vi "CD Read Engine_Parse Message.vi"(8 "Error (in)":errorcluster, 9 "Inline Status Channels Refs":T1[](array[typedef]) format="%.0x", 10 "Record []":T11[](array[typedef]) {"type" format="%04x"; "activity" format="%04x"; "error" format="%04x"; "cwd1" format="%04x"; "cwd2" format="%04x"; "swd1" format="%04x"; "swd2" format="%04x"; "data" format="%04x"}, 11 "RT Inline Data_Data Description_Channels":T2[](array[typedef]) {"Frame Drescriptors"."RT"."Status Channel Ref" format="%.0x"; "Frame Drescriptors"."RT"."Words Block Data Refs"."Data Reference" format="%.0x"; "Frame Drescriptors"."RT"."Timestamp Channel Data Reference" format="%.0x"; "Frame Drescriptors"."BC"."Status Channel Refs" format="%.0x"; "Frame Drescriptors"."BC"."Words Block Data Refs"."Data Reference" format="%.0x"; "Frame Drescriptors"."BC"."Timestamp Channel Data Reference" format="%.0x"}) -> (0 "Error (out)":errorcluster)   [LabVIEW 2020, in "Ballard MIL-1553 Engine.lvlib"]
uses:
  Ballard MIL-1553 Engine.lvlib
  <instrlib>/BTICardLib/Public/Controls/1553 Record.ctl
  Controls/RT Inline Data_Data Description_Channel.ctl
  Controls/RT Inline Frame Descriptor.ctl
  Controls/RT Inline Frame Descriptor_BC.ctl
  <vilib>/NI VeriStand/Custom Device API/Data Reference.ctl
  <vilib>/NI VeriStand/Custom Device API/Block Data Reference.ctl
  <vilib>/NI VeriStand/Custom Device API/Custom Device Item Ref.ctl
  Controls/RT Inline Frame Descriptor_RT.ctl
  Shared/Controls and Global/RT CWD2.ctl
  Shared/Controls and Global/RT CWD1.ctl
  Shared/Controls and Global/RT messageType.ctl
  <vilib>/NI VeriStand/Custom Device Tools/Custom Device Utility Library/Custom Device Utility Library.lvlib
  Shared/Ballard 1553 Shared.lvlib
  <vilib>/NI VeriStand/Custom Device API/Custom Device API.lvlib
  <instrlib>/BTICardLib/BTICardLV.lvlib
panel:
  out "Physical Channel":u16
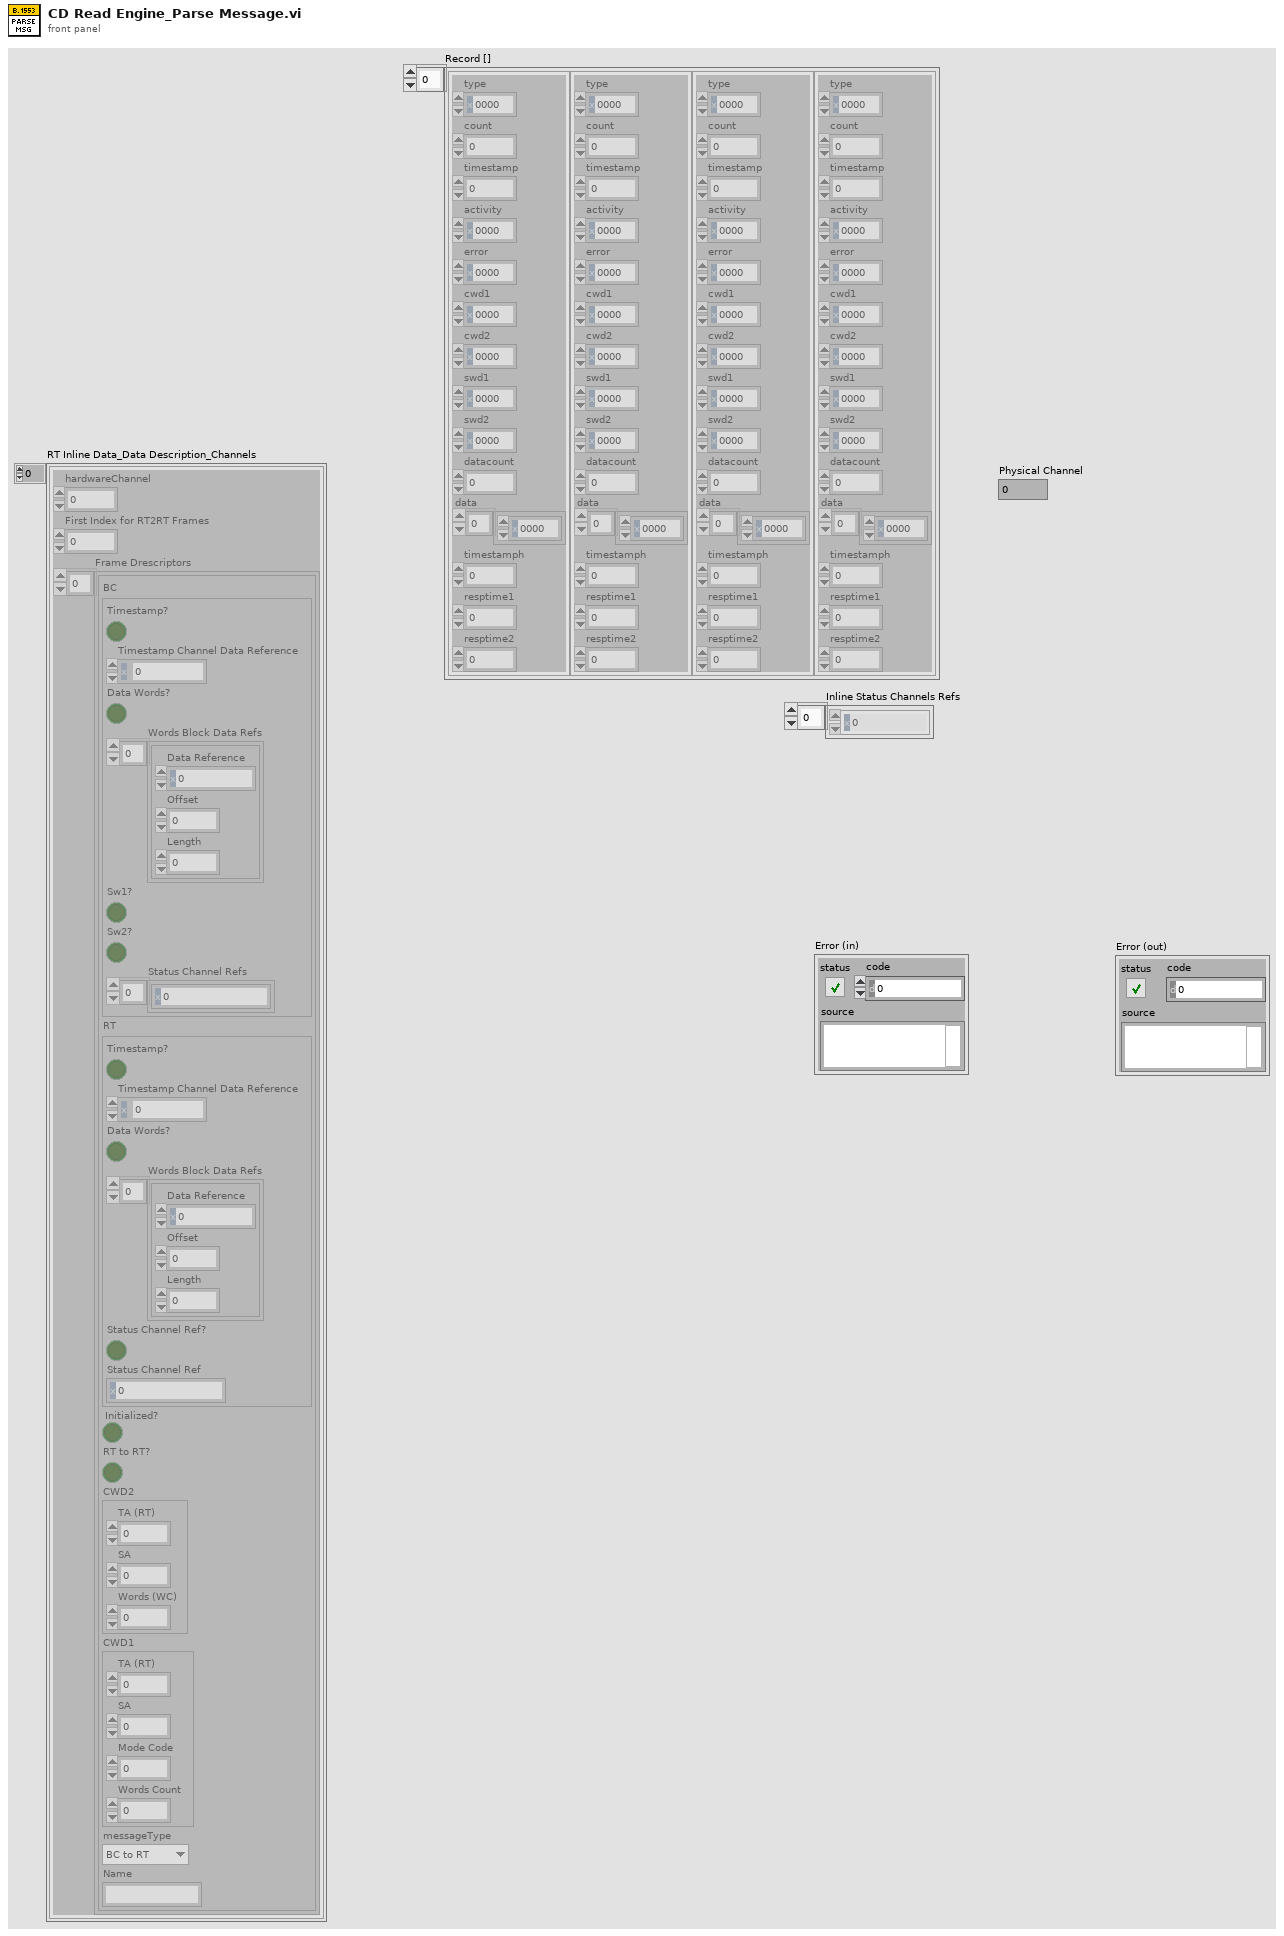
[diagram p1: front panel]
types:
  T1 = typedef "Custom Device API.lvlib/Data Reference.ctl" = i32
  T2 = typedef "Ballard MIL-1553 Engine.lvlib/RT Inline Data_Data Description_Channel.ctl" = cluster{"hardwareChannel":u16, "First Index for RT2RT Frames":i32, "Frame Drescriptors":T3[]}
  T3 = typedef "Ballard MIL-1553 Engine.lvlib/RT Inline Frame Descriptor.ctl" = cluster{"BC":T4, "RT":T7, "Initialized?":bool, "RT to RT?":bool, "CWD2":T8, "CWD1":T9, "messageType":T10, "Name":string}
  T4 = typedef "Ballard MIL-1553 Engine.lvlib/RT Inline Frame Descriptor_BC.ctl" = cluster{"Timestamp?":bool, "Timestamp Channel Data Reference":T1, "Data Words?":bool, "Words Block Data Refs":T5[], "Sw1?":bool, "Sw2?":bool, "Status Channel Refs":T6[]}
  T5 = typedef "Custom Device API.lvlib/Block Data Reference.ctl" = cluster{"Data Reference":T1, "Offset":u64, "Length":u64}
  T6 = typedef "Custom Device API.lvlib/Custom Device Item Ref.ctl" = u64
  T7 = typedef "Ballard MIL-1553 Engine.lvlib/RT Inline Frame Descriptor_RT.ctl" = cluster{"Timestamp?":bool, "Timestamp Channel Data Reference":T1, "Data Words?":bool, "Words Block Data Refs":T5[], "Status Channel Ref?":bool, "Status Channel Ref":T6}
  T8 = typedef "Ballard 1553 Shared.lvlib/RT CWD2.ctl" = cluster{"TA (RT)":i8, "SA":i8, "Words (WC)":i8}
  T9 = typedef "Ballard 1553 Shared.lvlib/RT CWD1.ctl" = cluster{"TA (RT)":i8, "SA":i8, "Mode Code":i8, "Words Count":i8}
  T10 = typedef "Ballard 1553 Shared.lvlib/RT messageType.ctl" = enum16{"BC to RT", "RT to BC", "RT to RT", "MC (Rx)", "MC (Tx)"}
  T11 = typedef "BTICardLV.lvlib/1553 Record.ctl" = cluster{"type":u16, "count":u16, "timestamp":u32, "activity":u16, "error":u16, "cwd1":u16, "cwd2":u16, "swd1":u16, "swd2":u16, "datacount":u16, "data":u16[], "timestamph":u32, "resptime1":u16, "resptime2":u16}
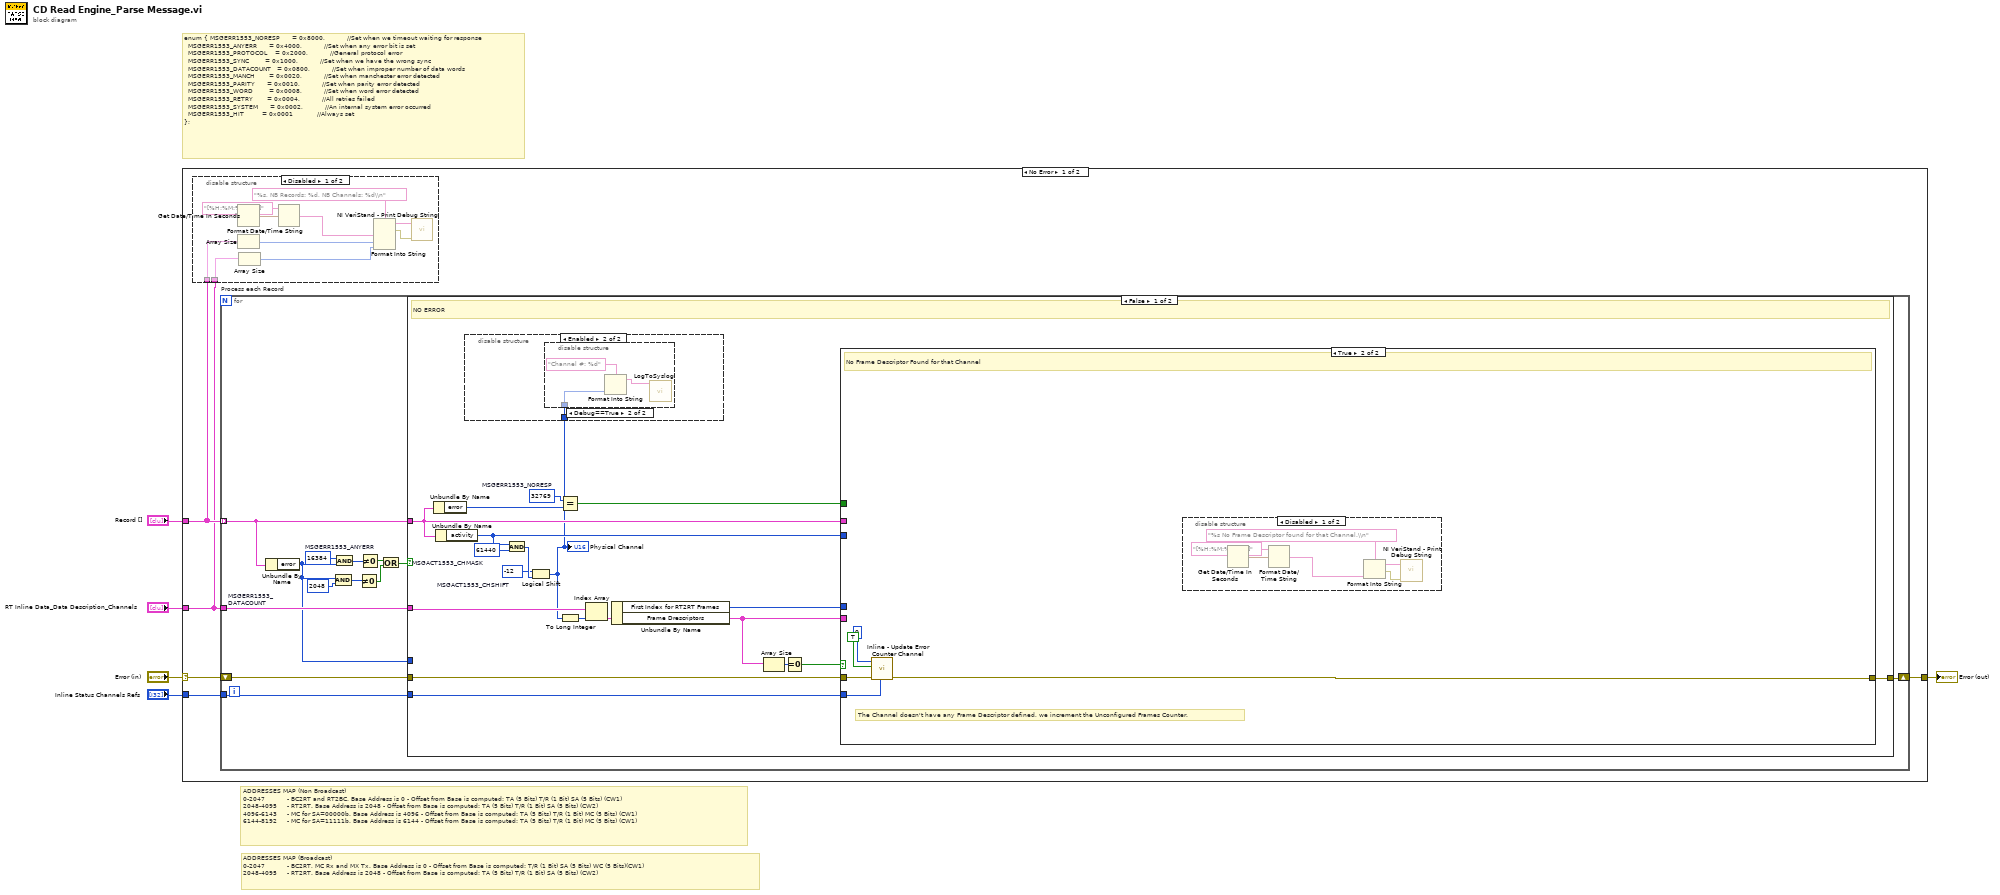
[diagram p0: block diagram]
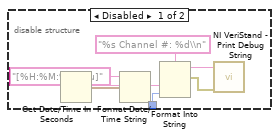
[diagram p2: hidden frame]
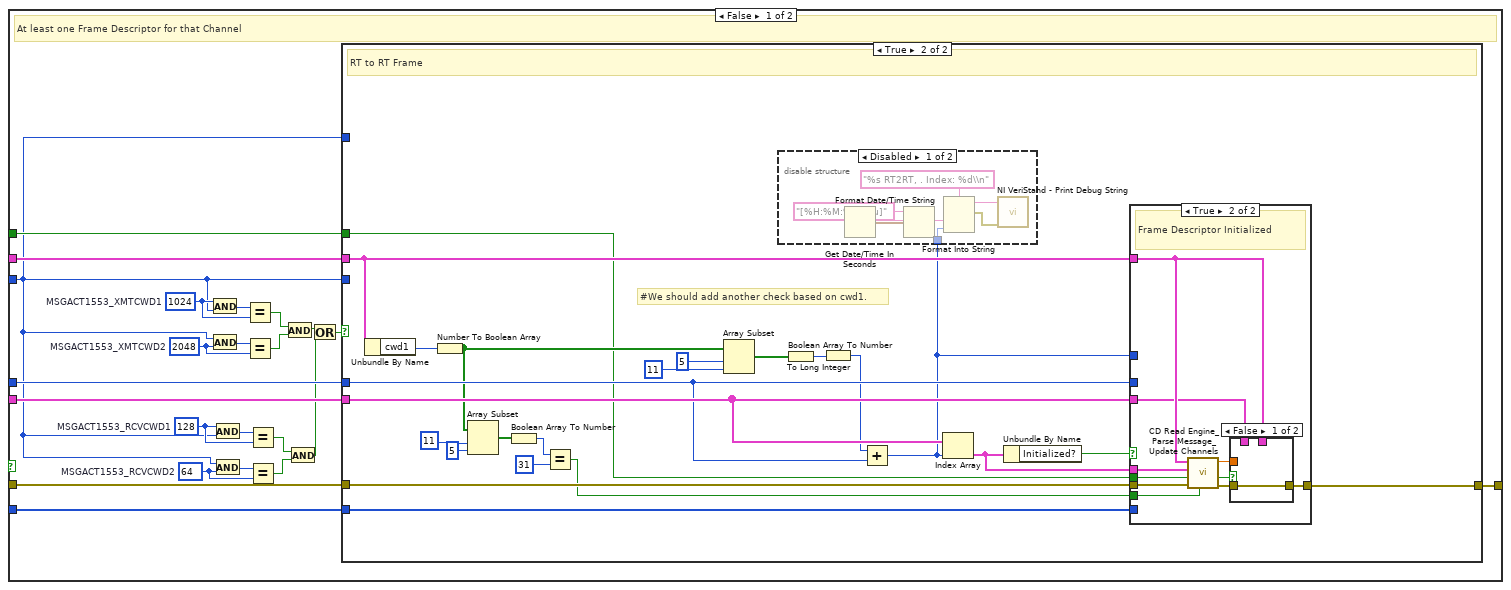
[diagram p4: hidden frame]
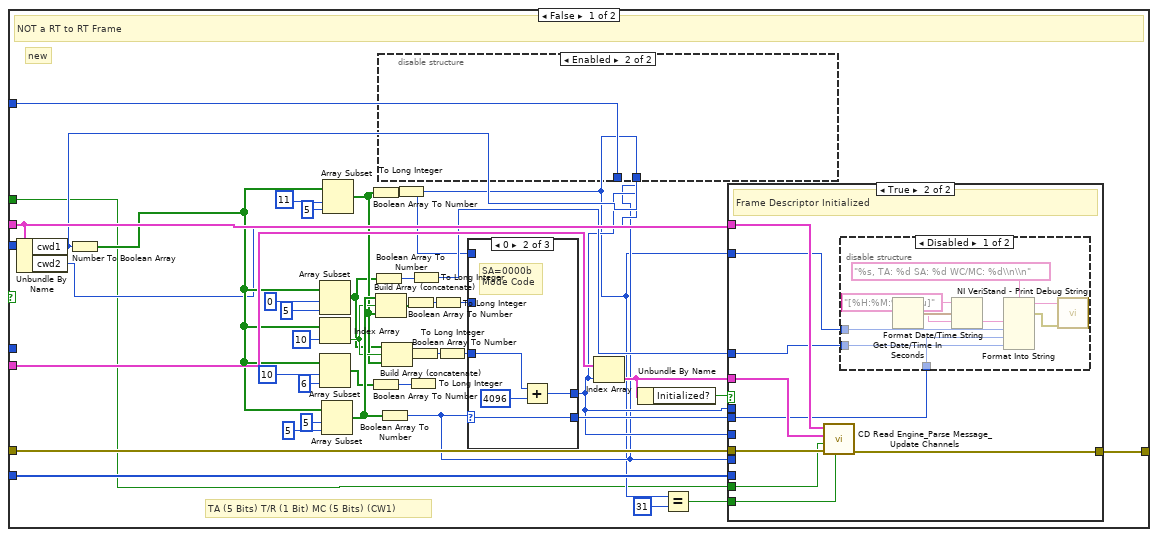
[diagram p5: hidden frame]
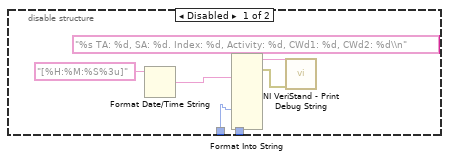
[diagram p6: hidden frame]
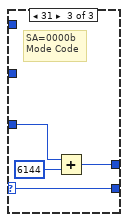
[diagram p8: hidden frame]
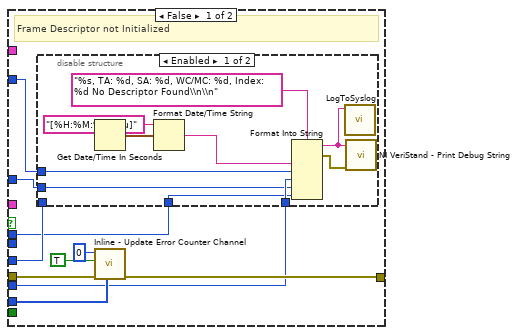
[diagram p9: hidden frame]
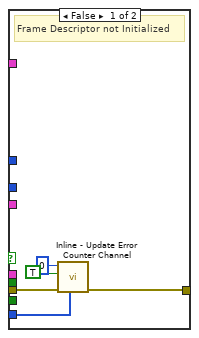
[diagram p13: hidden frame]
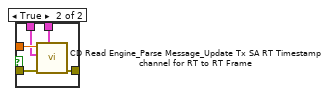
[diagram p14: hidden frame]
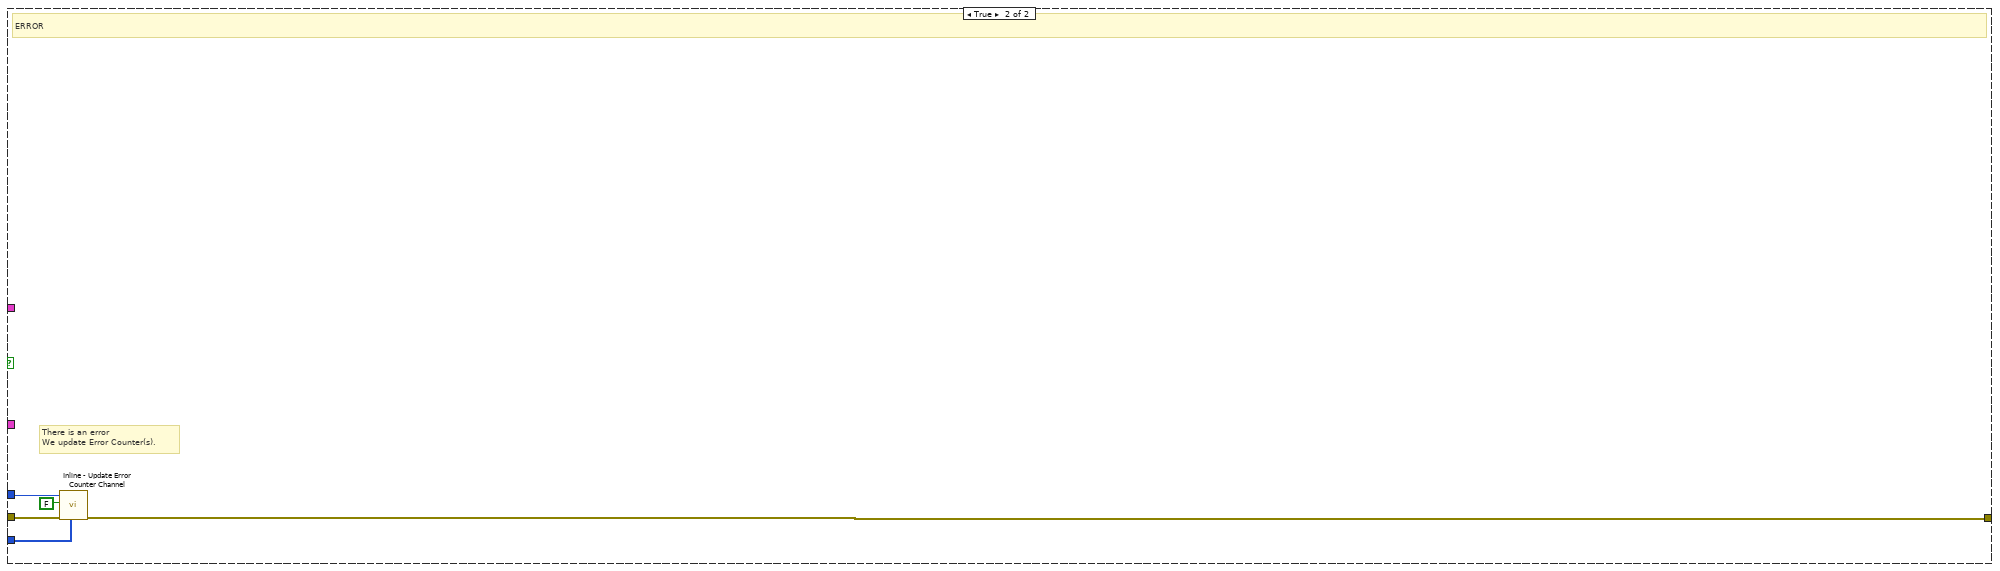
[diagram p16: hidden frame]
diagram:
  # "ADDRESSES MAP (Broadcast) \n0-2047           - BC2RT, MC Rx and MX Tx. Base Address is 0 - Offset from Base is computed: T/R (1 Bit) SA (5 Bits) WC (5 Bits)(CW1)\n2048-4095     - RT2RT. Base Address is 2048 - Offset from Base is computed: TA (5 Bits) T/R (1 Bit) SA (5 Bits) (CW2)"
  # "ADDRESSES MAP (Non Broadcast) \n0-2047           - BC2RT and RT2BC. Base Address is 0 - Offset from Base is computed: TA (5 Bits) T/R (1 Bit) SA (5 Bits) (CW1)\n2048-4095     - RT2RT. Base Address is 2048 - Offset from Base is computed: TA (5 Bits) T/R (1 Bit) SA (5 Bits) (CW2)\n4096-6143     - MC for SA=00000b. Base Address is 4096 - Offset from Base is computed: TA (5 Bits) T/R (1 Bit) MC (5 Bits) (CW1)\n6144-8192     - MC for SA=11111b. Base Address is 6144 - Offset from Base is computed: TA (5 Bits) T/R (1 Bit) MC (5 Bits) (CW1)"
  # "enum {\tMSGERR1553_NORESP      = 0x8000,           //Set when we timeout waiting for response\n\t\tMSGERR1553_ANYERR      = 0x4000,           //Set when any error bit is set\n\t\tMSGERR1553_PROTOCOL    = 0x2000,           //General protocol error\n\t\tMSGERR1553_SYNC        = 0x1000,           //Set when we have the wrong sync\n\t\tMSGERR1553_DATACOUNT   = 0x0800,           //Set when improper number of data words\n\t\tMSGERR1553_MANCH       = 0x0020,           //Set when manchester error detected\n\t\tMSGERR1553_PARITY      = 0x0010,           //Set when parity error detected\n\t\tMSGERR1553_WORD        = 0x0008,           //Set when word error detected\n\t\tMSGERR1553_RETRY       = 0x0004,           //All retries failed\n\t\tMSGERR1553_SYSTEM      = 0x0002,           //An internal system error occurred\n\t\tMSGERR1553_HIT         = 0x0001            //Always set\n};"
  n1 = case shown="No Error" "Error (in)" {
    selector: "Error (in)" -> [w9 w255]
    tunnel: "Record []" -> [w8 _]
    tunnel: [w10 w255] -> w4
    tunnel: "RT Inline Data_Data Description_Channels" -> [w6 _]
    tunnel: "Inline Status Channels Refs" -> [w7 _]
    frame No Error {
      n2 = disable-structure shown="Disabled" {
        disable-tunnel: w8 -> [w254 _]
        disable-tunnel: w6 -> [w246 _]
        frame Disabled {
          n3 = Get Date/Time In Seconds() -> (seconds since 1Jan1904=w253:timestamp)
          n4 = Array Size(array=w254) -> (size(s)=w251:i32)
          n5 = Array Size(array=w246) -> (size(s)=w245:i32)
          n6 = Format Date/Time String(time format string (%c)="[%H:%M:%S%3u]", seconds (now)=w253) -> (date/time string=w252:string)  [unwired: 1 in]
          n7 = Format Into String(format string="%s, NB Records: %d, NB Channels: %d\\n", w252, w251, w245) -> (resulting string=w247:string, error out=w248:errorcluster)  [unwired: 2 in]
          n8 = call <vilib>:"NI VeriStand - Print Debug String.vi"("error in (no error)"=w248, "Message"=w247) -> ()  [unwired: 9 in, 1 out]
        }
        frame Enabled {
        }
      }
      n9 = for "Process each Record" {
        tunnel: w8 -> [w23] mode=indexing
        shift-right: [w22] -> w10
        shift-left: w9 -> [w21]
        tunnel: w7 -> [w20]
        tunnel: w6 -> [w19]
        w11 = u16 2048  # MSGERR1553_DATACOUNT
        w18 = u16 16384  # MSGERR1553_ANYERR
        n10 = Unbundle By Name(w23) -> ("error"=w14:u16)
        n11 = And(x=w14, y=w11) -> (x .and. y?=w13:u16)
        n12 = And(x=w18, y=w14) -> (x .and. y?=w17:u16)
        n13 = Not Equal To 0?(x=w13) -> (x != 0?=w12:bool)
        n14 = Not Equal To 0?(x=w17) -> (x != 0?=w16:bool)
        n15 = Or(x=w16, y=w12) -> (x .or. y?=w15:bool)
        n16 = case "Channel Found?" shown="False" w15 {
          tunnel: w21 -> [w41 w243]
          tunnel: [w42 w241] -> w22
          tunnel: w23 -> [w29 _]
          tunnel: w20 -> [w32 w242]
          tunnel: w19 -> [w39 _]
          tunnel: w14 -> [_ w244]
          frame False {
            w27 = u16 32769  # MSGERR1553_NORESP
            w30 = i16 -12  # MSGACT1553_CHSHIFT
            w40 = u16 61440  # MSGACT1553_CHMASK
            # "NO ERROR"
            n17 = Unbundle By Name(w29) -> ("error"=w28:u16)
            n18 = Unbundle By Name(w29) -> ("activity"=w34:u16)
            n19 = And(x=w34, y=w40) -> (x .and. y?=w31:u16)
            n20 = Logical Shift(y=w30, x=w31) -> (x << y=w25:u16)
            "Physical Channel" <- w25
            n21 = disable-structure shown="Enabled" {
              disable-tunnel: w25 -> [w43 w50]
              frame Disabled {
                n22 = Get Date/Time In Seconds() -> (seconds since 1Jan1904=w49:timestamp)
                n23 = Format Date/Time String(time format string (%c)="[%H:%M:%S%3u]", seconds (now)=w49) -> (date/time string=w48:string)  [unwired: 1 in]
                n24 = Format Into String(format string="%s Channel #: %d\\n", w48, w43) -> (resulting string=w44:string, error out=w45:errorcluster)  [unwired: 2 in]
                n25 = call <vilib>:"NI VeriStand - Print Debug String.vi"("error in (no error)"=w45, "Message"=w44) -> ()  [unwired: 9 in, 1 out]
              }
              frame Enabled {
                n26 = disable-structure shown="Debug==True" {
                  disable-tunnel: w50 -> [_ w52]
                  frame condition #0 (active) {
                  }
                  frame condition #1 {
                    n27 = Format Into String(format string="Channel #: %d", w52) -> (resulting string=w51:string)  [unwired: 2 in, 1 out]
                    n28 = call "LogToSyslog.vi"("message"=w51) -> ()  [unwired: 9 in, 2 out]
                  }
                }
              }
            }
            n29 = Equal?(x=w27, y=w28) -> (x = y?=w26:bool)
            n30 = To Long Integer(number=w25) -> (32bit integer=w38:i32)
            n31 = Index Array(array=w39, index=w38) -> (element=w36:T2)
            n32 = Unbundle By Name(w36) -> ("First Index for RT2RT Frames"=w33:i32, "Frame Drescriptors"=w35:T3[])
            n33 = Array Size(array=w35) -> (size(s)=w37:i32)
            n34 = Equal To 0?(x=w37) -> (x = 0?=w24:bool)
            n35 = case shown="True" w24 {
              tunnel: [w76 w229] -> w42
              tunnel: w29 -> [w75 _]
              tunnel: w41 -> [w74 w232]
              tunnel: w35 -> [w67 _]
              tunnel: w34 -> [w54 _]
              tunnel: w33 -> [w68 _]
              tunnel: w32 -> [w66 w231]
              tunnel: w26 -> [w64 _]
              frame False {
                w63 = u16 128  # MSGACT1553_RCVCWD1
                w62 = u16 64  # MSGACT1553_RCVCWD2
                w65 = u16 1024  # MSGACT1553_XMTCWD1
                w69 = u16 2048  # MSGACT1553_XMTCWD2
                # "At least one Frame Descriptor for that Channel"
                n36 = And(x=w65, y=w54) -> (x .and. y?=w72:u16)
                n37 = And(x=w54, y=w69) -> (x .and. y?=w70:u16)
                n38 = And(x=w63, y=w54) -> (x .and. y?=w59:u16)
                n39 = And(x=w54, y=w62) -> (x .and. y?=w61:u16)
                n40 = Equal?(x=w72, y=w65) -> (x = y?=w73:bool)
                n41 = Equal?(x=w70, y=w69) -> (x = y?=w71:bool)
                n42 = Equal?(x=w59, y=w63) -> (x = y?=w58:bool)
                n43 = Equal?(x=w61, y=w62) -> (x = y?=w60:bool)
                n44 = And(x=w73, y=w71) -> (x .and. y?=w56:bool)
                n45 = And(x=w58, y=w60) -> (x .and. y?=w55:bool)
                n46 = Or(x=w56, y=w55) -> (x .or. y?=w57:bool)
                n47 = case shown="True" w57 {
                  tunnel: w75 -> [w116 w195]
                  tunnel: w74 -> [w117 w199]
                  tunnel: [w118 w200] -> w76
                  tunnel: w68 -> [_ w196]
                  tunnel: w67 -> [w115 w198]
                  tunnel: w66 -> [w114 w197]
                  tunnel: w64 -> [w77 w179]
                  tunnel: w54 -> [_ _]
                  tunnel: w54 -> [w113 _]
                  frame False {
                    # "TA (5 Bits) T/R (1 Bit) MC (5 Bits) (CW1)"
                    # "new"
                    # "NOT a RT to RT Frame"
                    n48 = Unbundle By Name(w116) -> ("cwd1"=w111:u16, "cwd2"=w110:u16)
                    n49 = Number To Boolean Array(number=w111) -> (Boolean array=w112:bool[])
                    n50 = Array Subset(array=w112, index=0, length=5) -> (w85:bool[])
                    n51 = Index Array(array=w112, index=10) -> (element=w88:bool)
                    n52 = Array Subset(array=w112, index=10, length=6) -> (w83:bool[])
                    n53 = Array Subset(array=w112, index=5, length=5) -> (w89:bool[])
                    n54 = Array Subset(array=w112, index=11, length=5) -> (w87:bool[])
                    n55 = Boolean Array To Number(Boolean array=w87) -> (number=w94:u32)
                    n56 = Boolean Array To Number(Boolean array=w83) -> (number=w84:u32)
                    n57 = Boolean Array To Number(Boolean array=w85) -> (number=w98:u32)
                    n58 = Build Array (concatenate)(w89, w88, w87) -> (w103:bool[])
                    n59 = Boolean Array To Number(Boolean array=w89) -> (number=w81:u16)
                    n60 = Build Array (concatenate)(w85, w88, w87) -> (w86:bool[])
                    n61 = To Long Integer(number=w94) -> (32bit integer=w80:i32)
                    n62 = Boolean Array To Number(Boolean array=w103) -> (number=w100:u16)
                    n63 = To Long Integer(number=w84) -> ()  [unwired: 1 out]
                    n64 = Boolean Array To Number(Boolean array=w86) -> (number=w91:u16)
                    n65 = To Long Integer(number=w98) -> (32bit integer=w97:i32)
                    n66 = To Long Integer(number=w100) -> (32bit integer=w93:i32)
                    n67 = To Long Integer(number=w91) -> (32bit integer=w90:i32)
                    n68 = case shown="0" w81 {
                      selector: w81 -> [w131 w133 w137]
                      tunnel: w80 -> [_ _ _]
                      tunnel: [w130 w135 w139] -> w82
                      tunnel: w93 -> [w130 _ _]
                      tunnel: [w131 w133 w137] -> w99
                      tunnel: w90 -> [_ w132 w136]
                      frame 1, Default {
                      }
                      frame 0 {
                        # "SA=0000b\nMode Code"
                        n69 = Add(x=w132, y=4096) -> (x+y=w135:i32)
                      }
                      frame 31 {
                        # "SA=0000b\nMode Code"
                        n70 = Add(x=w136, y=6144) -> (x+y=w139:i32)
                      }
                    }
                    n71 = disable-structure shown="Enabled" {
                      disable-tunnel: w80 -> [w125 _]
                      disable-tunnel: w82 -> [w124 _]
                      disable-tunnel: w81 -> [w122 _]
                      disable-tunnel: w113 -> [w121 _]
                      disable-tunnel: w111 -> [w120 _]
                      disable-tunnel: w110 -> [w119 _]
                      frame Disabled {
                        n72 = Format Date/Time String(time format string (%c)="[%H:%M:%S%3u]") -> (date/time string=w129:string)  [unwired: 2 in]
                        n73 = Format Into String(format string="%s TA: %d, SA: %d. Index: %d, Activity: %d, CWd1: %d, CWd2: %d\\n", w129, w125, w122, w124, w121, w120, w119) -> (resulting string=w126:string, error out=w127:errorcluster)  [unwired: 2 in]
                        n74 = call <vilib>:"NI VeriStand - Print Debug String.vi"("error in (no error)"=w127, "Message"=w126) -> ()  [unwired: 9 in, 1 out]
                      }
                      frame Enabled {
                      }
                    }
                    n75 = Index Array(array=w115, index=w82) -> (element=w109:T3)
                    n76 = Unbundle By Name(w109) -> ("Initialized?"=w108:bool)
                    n77 = Equal?(x=w80, y=31) -> (x = y?=w78:bool)
                    n78 = case shown="True" w108 {
                      tunnel: [w146 w168] -> w118
                      tunnel: w117 -> [w147 w167]
                      tunnel: w116 -> [_ w166]
                      tunnel: w109 -> [_ w165]
                      tunnel: w114 -> [w145 _]
                      tunnel: w80 -> [w144 w164]
                      tunnel: w99 -> [_ w163]
                      tunnel: w97 -> [w141 w162]
                      tunnel: w82 -> [w143 _]
                      tunnel: w81 -> [w142 _]
                      tunnel: w82 -> [w140 _]
                      tunnel: w78 -> [_ w160]
                      tunnel: w77 -> [_ w161]
                      frame False {
                        # "Frame Descriptor not Initialized"
                        n79 = disable-structure shown="Enabled" {
                          disable-tunnel: w144 -> [w154 _]
                          disable-tunnel: w143 -> [_ _]
                          disable-tunnel: w142 -> [w153 _]
                          disable-tunnel: w141 -> [w152 _]
                          disable-tunnel: w140 -> [w151 _]
                          frame Enabled {
                            n80 = Get Date/Time In Seconds() -> (seconds since 1Jan1904=w159:timestamp)
                            n81 = Format Date/Time String(time format string (%c)="[%H:%M:%S%3u]", seconds (now)=w159) -> (date/time string=w158:string)  [unwired: 1 in]
                            n82 = Format Into String(format string="%s, TA: %d, SA: %d, WC/MC: %d, Index: %d No Descriptor Found\\n\\n", w158, w154, w153, w152, w151) -> (resulting string=w150:string, error out=w155:errorcluster)  [unwired: 2 in]
                            n83 = call "LogToSyslog.vi"("message"=w150) -> ()  [unwired: 9 in, 2 out]
                            n84 = call <vilib>:"NI VeriStand - Print Debug String.vi"("error in (no error)"=w155, "Message"=w150) -> ()  [unwired: 9 in, 1 out]
                          }
                          frame Disabled {
                          }
                        }
                        n85 = call "Inline - Update Error Counter Channel.vi"("Inline Status Channels Refs"=w145, "error in (no error)"=w147, "Increment Unconfigured Frames Counter?"=TRUE, "error"=u16 0) -> ("error IO"=w146:errorcluster)  [unwired: 6 in, 1 out]
                      }
                      frame True {
                        # "Frame Descriptor Initialized"
                        n86 = call "CD Read Engine_Parse Message_Update Channels.vi"("Broadcast?"=w160, "error in (no error)"=w167, "NORESP?"=w161, "Frame Descriptor"=w165, "record in"=w166) -> ("error out"=w168:errorcluster)  [unwired: 4 in, 2 out]
                        n87 = disable-structure shown="Disabled" {
                          disable-tunnel: w164 -> [w171 _]
                          disable-tunnel: w163 -> [w170 _]
                          disable-tunnel: w162 -> [w169 _]
                          frame Disabled {
                            n88 = Get Date/Time In Seconds() -> (seconds since 1Jan1904=w177:timestamp)
                            n89 = Format Date/Time String(time format string (%c)="[%H:%M:%S%3u]", seconds (now)=w177) -> (date/time string=w176:string)  [unwired: 1 in]
                            n90 = Format Into String(format string="%s, TA: %d SA: %d WC/MC: %d\\n\\n", w176, w171, w170, w169) -> (resulting string=w172:string, error out=w173:errorcluster)  [unwired: 2 in]
                            n91 = call <vilib>:"NI VeriStand - Print Debug String.vi"("error in (no error)"=w173, "Message"=w172) -> ()  [unwired: 9 in, 1 out]
                          }
                          frame Enabled {
                          }
                        }
                      }
                    }
                  }
                  frame True {
                    # "#We should add another check based on cwd1."
                    # "RT to RT Frame"
                    n92 = Unbundle By Name(w195) -> ("cwd1"=w192:u16)
                    n93 = Number To Boolean Array(number=w192) -> (Boolean array=w185:bool[])
                    n94 = Array Subset(array=w185, index=11, length=5) -> (w181:bool[])
                    n95 = Boolean Array To Number(Boolean array=w181) -> (number=w180:u32)
                    n96 = Equal?(x=w180, y=u32 31) -> (x = y?=w178:bool)
                    n97 = Array Subset(array=w185, index=5, length=11) -> (w191:bool[])
                    n98 = Boolean Array To Number(Boolean array=w191) -> (number=w190:u32)
                    n99 = To Long Integer(number=w190) -> (32bit integer=w189:i32)
                    n100 = Add(x=w189, y=w196) -> (x+y=w187:i32)
                    n101 = disable-structure shown="Disabled" {
                      disable-tunnel: w187 -> [w201 _]
                      frame Disabled {
                        n102 = Get Date/Time In Seconds() -> (seconds since 1Jan1904=w207:timestamp)
                        n103 = Format Date/Time String(time format string (%c)="[%H:%M:%S%3u]", seconds (now)=w207) -> (date/time string=w206:string)  [unwired: 1 in]
                        n104 = Format Into String(format string="%s RT2RT, . Index: %d\\n", w206, w201) -> (resulting string=w202:string, error out=w203:errorcluster)  [unwired: 2 in]
                        n105 = call <vilib>:"NI VeriStand - Print Debug String.vi"("error in (no error)"=w203, "Message"=w202) -> ()  [unwired: 9 in, 1 out]
                      }
                      frame Enabled {
                      }
                    }
                    n106 = Index Array(array=w198, index=w187) -> (element=w188:T3)
                    n107 = Unbundle By Name(w188) -> ("Initialized?"=w186:bool)
                    n108 = case shown="True" w186 {
                      tunnel: [w209 w218] -> w200
                      tunnel: w199 -> [w210 w222]
                      tunnel: w195 -> [_ w220]
                      tunnel: w188 -> [_ w221]
                      tunnel: w197 -> [w208 _]
                      tunnel: w187 -> [_ _]
                      tunnel: w179 -> [_ w215]
                      tunnel: w198 -> [_ w216]
                      tunnel: w196 -> [_ _]
                      tunnel: w178 -> [_ w214]
                      frame False {
                        # "Frame Descriptor not Initialized"
                        n109 = call "Inline - Update Error Counter Channel.vi"("Inline Status Channels Refs"=w208, "error in (no error)"=w210, "Increment Unconfigured Frames Counter?"=TRUE, "error"=u16 0) -> ("error IO"=w209:errorcluster)  [unwired: 6 in, 1 out]
                      }
                      frame True {
                        # "Frame Descriptor Initialized"
                        n110 = call "CD Read Engine_Parse Message_Update Channels.vi"("Broadcast?"=w214, "error in (no error)"=w222, "NORESP?"=w215, "Frame Descriptor"=w221, "record in"=w220) -> ("error out"=w219:errorcluster, "Valid Frame?"=w213:bool, "Timestamp (s)"=w217:dbl)  [unwired: 4 in]
                        n111 = case shown="False" w213 {
                          tunnel: w220 -> [_ w228]
                          tunnel: w219 -> [w223 w227]
                          tunnel: [w223 w226] -> w218
                          tunnel: w217 -> [_ w225]
                          tunnel: w216 -> [_ w224]
                          frame False {
                          }
                          frame True {
                            n112 = call "CD Read Engine_Parse Message_Update Tx SA RT Timestamp channel for RT to RT Frame.vi"("record in"=w228, "error in (no error)"=w227, "Frame Drescriptors"=w224, "Timestamp (s)"=w225) -> ("error out"=w226:errorcluster)  [unwired: 7 in]
                          }
                        }
                      }
                    }
                  }
                }
              }
              frame True {
                # "The Channel doesn't have any Frame Descriptor defined, we increment the Unconfigured Frames Counter."
                # "No Frame Descriptor Found for that Channel"
                n113 = call "Inline - Update Error Counter Channel.vi"("Inline Status Channels Refs"=w231, "error in (no error)"=w232, "Increment Unconfigured Frames Counter?"=TRUE, "error"=u16 0) -> ("error IO"=w229:errorcluster)  [unwired: 6 in, 1 out]
                n114 = disable-structure shown="Disabled" {
                  frame Disabled {
                    n115 = Get Date/Time In Seconds() -> (seconds since 1Jan1904=w239:timestamp)
                    n116 = Format Date/Time String(time format string (%c)="[%H:%M:%S%3u]", seconds (now)=w239) -> (date/time string=w238:string)  [unwired: 1 in]
                    n117 = Format Into String(format string="%s No Frame Descriptor found for that Channel.\\n", w238) -> (resulting string=w234:string, error out=w235:errorcluster)  [unwired: 2 in]
                    n118 = call <vilib>:"NI VeriStand - Print Debug String.vi"("error in (no error)"=w235, "Message"=w234) -> ()  [unwired: 9 in, 1 out]
                  }
                  frame Enabled {
                  }
                }
              }
            }
          }
          frame True {
            # "There is an error\nWe update Error Counter(s)."
            # "ERROR"
            n119 = call "Inline - Update Error Counter Channel.vi"("Inline Status Channels Refs"=w242, "error in (no error)"=w243, "Increment Unconfigured Frames Counter?"=FALSE, "error"=w244) -> ("error IO"=w241:errorcluster)  [unwired: 6 in, 1 out]
          }
        }
      }
    }
    frame Error {
    }
  }
  "Error (out)" <- w4
